vi "QX_Connect Device.vi"(8 "error in":errorcluster, 11 "Devices":refnum<k24>[](array[refnum])) -> (0 "error out":errorcluster, 1 "Connect?":bool, 3 "Devices":refnum<k24>[](array[refnum]))   [LabVIEW 2016]
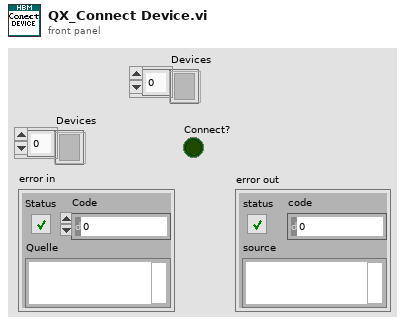
[diagram p1: front panel]
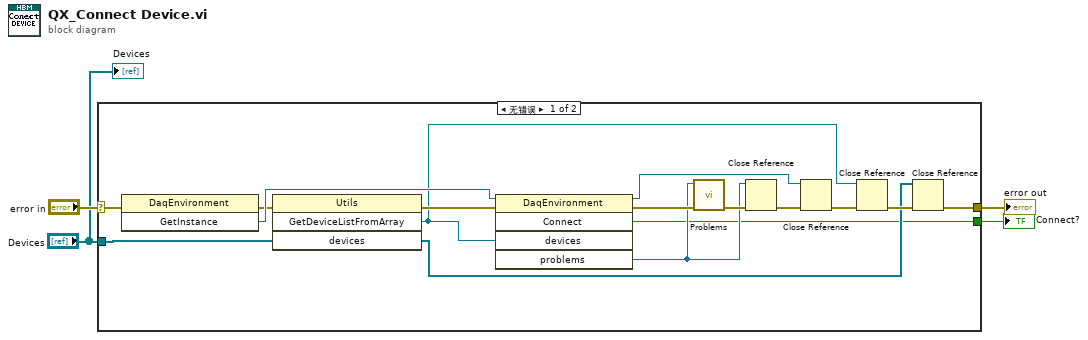
[diagram p0: block diagram]
diagram:
  n1 = case shown="无错误" "error in" {
    selector: "error in" -> [w20 w21]
    tunnel: [w5 w21] -> w3
    tunnel: "Devices" -> [w6 _]
    tunnel: [w7 _] -> w2
    frame No Error {
      n2 = invoke on="Methodenknoten" class="DaqEnvironment" method="GetInstance"(error in=w20) -> (error out=w16:errorcluster, "GetInstance"=w17:refnum<k24>)  [unwired: 2 in, 1 out]
      n3 = invoke on="Methodenknoten" class="Utils" method="GetDeviceListFromArray"(error in=w16, "devices"=w6) -> (error out=w19:errorcluster, "GetDeviceListFromArray"=w10:refnum<k24>, "devices"=w8:refnum<k24>[])  [unwired: 2 in, 1 out]
      n4 = invoke class="DaqEnvironment" method="Connect"(reference=w17, error in=w19, "devices"=w10) -> (reference out=w15:refnum<k24>, error out=w18:errorcluster, "Connect"=w7:bool, "problems"=w12:refnum<k24>)  [unwired: 2 in, 1 out]
      n5 = call "Problems.vi"("Error in"=w18, "Problems"=w12) -> ("Error out"=w13:errorcluster)  [unwired: 9 in]
      n6 = Close Reference(reference=w12, error in (no error)=w13) -> (error out=w14:errorcluster)
      n7 = Close Reference(reference=w15, error in (no error)=w14) -> (error out=w11:errorcluster)
      n8 = Close Reference(reference=w10, error in (no error)=w11) -> (error out=w9:errorcluster)
      n9 = Close Reference(reference=w8, error in (no error)=w9) -> (error out=w5:errorcluster)
    }
    frame Error {
    }
  }
  "error out" <- w3
  "Connect?" <- w2
  "Devices" <- "Devices"
